vi "Actor Core.vi"(8 "error in":errorcluster, 11 "Display Console in":refnum<class "Display Console.lvclass">) -> (0 "error out":errorcluster, 3 "Actor out":refnum<class "Actor.lvclass">)   [LabVIEW 2019, in "Display Console Actor.lvlib" / "Display Console.lvclass"]
doc: "(<B>Filename</B>: Actor Framework.lvlib:Actor.lvclass:Actor Core.vi)\n\nReceives messages to the actor, reacts to them, and initiates any error handling that may shut the actor down.\n\nDescendant classes may override this VI to append parallel tasks for the actor to complete while it handles messages. Overrides use the Call Parent Method node."
uses:
  Display Console.lvclass
  <vilib>/ActorFramework/Stop Msg/Stop Msg.lvclass
  <vilib>/ActorFramework/Actor/Actor.lvclass
  Abstract Display Console Actor/Abstract Display Console Actor/Abstract Display Console.lvclass
  C:/Workspace/CLA/Elevator AF/Abstract Display Console Actor/Abstract Display Console Actor/Abstract Display Console.lvclass
  C:/Program Files (x86)/National Instruments/LabVIEW 2019/vi.lib/ActorFramework/Actor/Actor.lvclass
  Elevator Direction.ctl
panel:
  out "Emergency":bool
  out "Door Open":bool
  out "Elevator Direction":T1
  out "Elevator Location":string
  out "Timing":dbl format="%#2.2g"
  # "[Covers: UI1]"
  # "[Covers: UI3C]"
  # "[Covers: UI3] \n[Covers: UI3A] \n[Covers: UI3A1] \n[Covers: UI3A2]"
  # "[Covers: UI3D] \n[Covers: UI3D1] \n[Covers: UI3D2]"
  # "[Covers: UI3B]"
  # "[Covers: UI3E]"
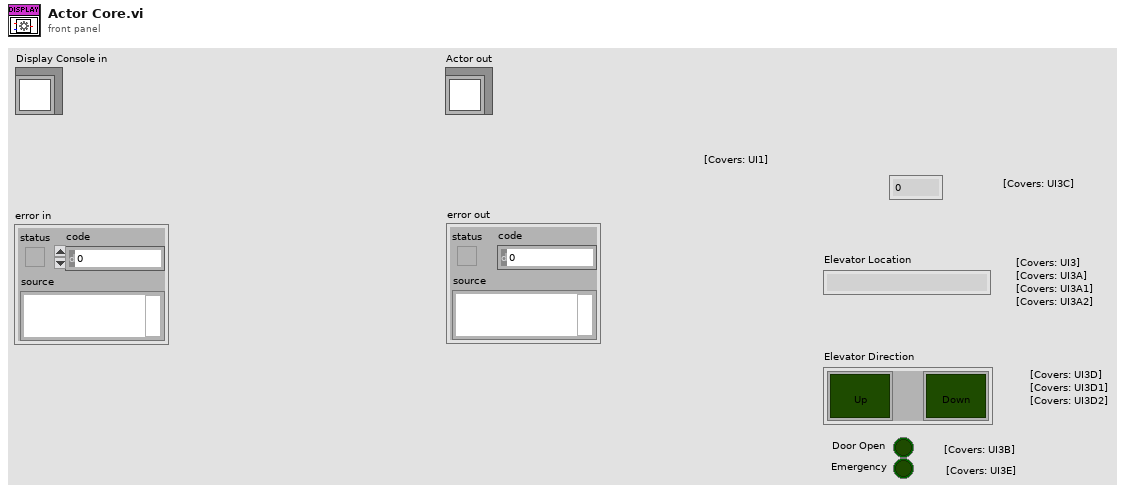
[diagram p1: front panel]
types:
  T1 = typedef "Display Console Actor.lvlib/Display Console.lvclass/Elevator Direction.ctl" = cluster{"Up":bool, "Down":bool}
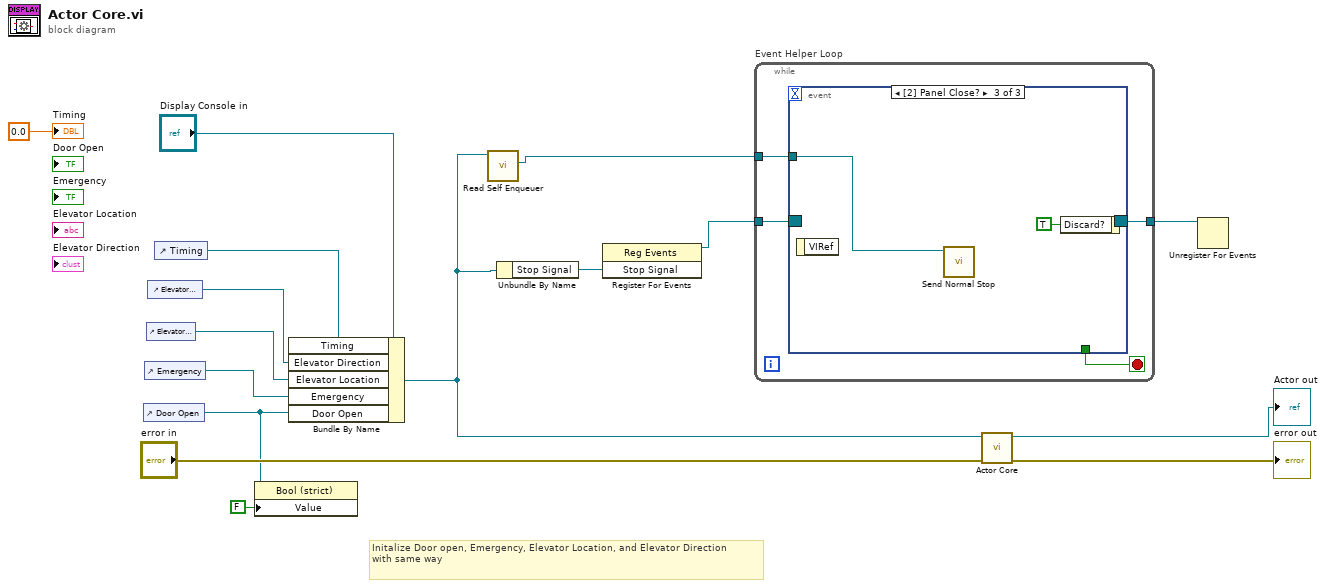
[diagram p0: block diagram]
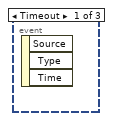
[diagram p2: hidden frame]
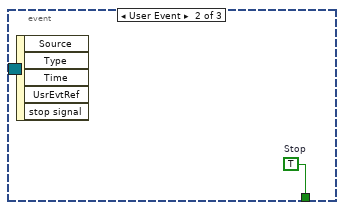
[diagram p3: hidden frame]
diagram:
  # "Initalize Door open, Emergency, Elevator Location, and Elevator Direction \nwith same way"
  n1 = control-ref of="Door Open"() -> (w6:refnum<vi>)
  n2 = control-ref of="Emergency"() -> (w4:refnum<vi>)
  n3 = control-ref of="Elevator Location"() -> (w3:refnum<vi>)
  n4 = control-ref of="Elevator Direction"() -> (w2:refnum<vi>)
  n5 = control-ref of="Timing"() -> (w1:refnum<vi>)
  n6 = property class="Bool (strict)"(reference=w6, "Value"=FALSE) -> ()  [unwired: 1 in, 2 out]
  n7 = Bundle By Name(cluster="Display Console in", "Timing"=w1, "Elevator Direction"=w2, "Elevator Location"=w3, "Emergency"=w4, "Door Open"=w6) -> (w7:refnum<class "Display Console.lvclass">)
  n8 = call <vilib>:"Read Self Enqueuer.vi"("Actor"=w7) -> ("Self Enqueuer"=w10:refnum<class "Message Enqueuer.lvclass">)  [unwired: 10 in]
  n9 = Unbundle By Name(w7) -> ("Stop Signal"=w13:refnum<user-event>)
  n10 = register-events(w13) -> (reference out=w12:refnum<event-registration>)  [unwired: 2 in, 1 out]
  n11 = while "Event Helper Loop" {
    tunnel: w10 -> [w20]
    tunnel: w12 -> [w19]
    tunnel: [w18] -> w11
    stop <- w17 stop-if-true
    n12 = event shown="[2] Panel Close?" {
      selector: w19 -> [_ _ _]
      dyn-events: [_ _ _] -> w18
      timeout: _ -> [_ _ _]
      tunnel: w20 -> [_ _ w23]
      tunnel: [_ w21 _] -> w17
      event Timeout {
        n13 = event-data() -> ()  [unwired: 1 in, 3 out]
      }
      event User Event {
        w21 = TRUE  # Stop
        n14 = event-data() -> ()  [unwired: 1 in, 5 out]
      }
      event Panel Close? {
        n15 = event-data() -> ()  [unwired: 1 in, 1 out]
        n16 = call <vilib>:"Send Normal Stop.vi"("Message Enqueuer"=w23) -> ()  [unwired: 10 in, 1 out]
        n17 = event-data("Discard?"=TRUE) -> ()  [unwired: 1 in, 1 out]
      }
    }
  }
  n18 = call-parent "Actor Core.vi"("error in"="error in", "Actor in"=w7) -> ("error out"=→"error out":errorcluster, "Actor out"=→"Actor out":refnum<class "Actor.lvclass">)  [unwired: 8 in]
  n19 = Unregister For Events(event registration refnum=w11) -> ()  [unwired: 1 in, 1 out]
  "Timing" <- 0.0 ("Timing")
